vi "ble_evt_gap_scan_response.vi"(8 "error in (no error)":errorcluster, 11 "COM Bluegiga in":refnum<visa-resource-name>) -> (0 "error out":errorcluster, 2 "Scan Response 1 Device":string[](array[string]), 3 "COM Bluegiga out":refnum<visa-resource-name>)   [LabVIEW 2017]
uses:
  type_def/message_type.ctl
  type_def/message_class.ctl
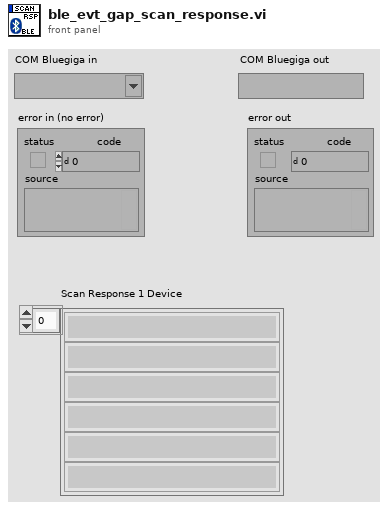
[diagram p1: front panel]
types:
  T1 = typedef "message_class.ctl" = u8
  T2 = typedef "message_type.ctl" = u8
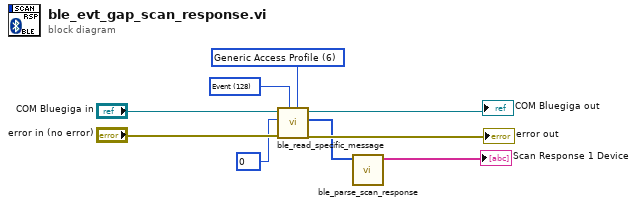
[diagram p0: block diagram]
diagram:
  w6 = T1 6 items=["System", "Persistent Store", "Attribute database", "Connection", "Attribute client", "Security Manager", "Generic Access Profile", "Hardware"] ("Command Class (System)")
  w7 = T2 128 items=["Command / Response"=0, "Event"=128] ("Message Type (Response)")
  n1 = call "ble_read_specific_message.vi"("Command Class (System)"=w6, "Message Type (Response)"=w7, "error in (no error)"="error in (no error)", "Message ID (0x00)"=u8 0, "COM Bluegiga in"="COM Bluegiga in") -> ("error out"=→"error out":errorcluster, "specific payload"=w2:u8[], "COM Bluegiga out"=→"COM Bluegiga out":refnum<visa-resource-name>)  [unwired: 2 in, 2 out]
  n2 = call "ble_parse_scan_response.vi"("Scan Response Data"=w2) -> ("Array Scan Response"=→"Scan Response 1 Device":string[])  [unwired: 10 in]
